vi "PRIME Detector Check Files and Add FITS data.vi"(5 "Observation":T2={"Priority"=0, "ID"="", "Observer"="", "Obj Name"="", "Obj Type"="", "RA and DEC String"={"RA"="HH:MM:SS.nnn", "DEC"="DEG:arcmin:arcsec.nn"}, "Filters"=[], "Integration Time"=0.0, "Observation Status"=enum."Error", "Offsets"={"RA"=0.0, "DEC"=0.0, "ROT"=0.0}, "Images"=0, "Dither Options"={"Dither"=enum."None", "Dither Radius"=0.0, "Dither Points"=0, "Dither Phase"=0.0, "B Offset"={"RA"=0.0, "DEC"=0.0}}, "Comment 1"="", "Comment 2"=""}, 7 "Detector Config":T8={"Detector"=0, "Offsets"=[[0, 0, 0, 0, 0, 0, 0, 0, 0, 0, 0, 0, 0, 0, 0, 0, 0, 0, 0, 0, 0, 0, 0, 0, 0, 0, 0, 0, 0, 0, 0, 0]], "Detector Computer"={"Machine"="192.168.121.11", "Password"="rSL!nux23456", "FITS File Path"="", "Port"=44444, "Header Path"="", "Name"=""}, "FITS hdr template0"=path "", "FITS hdr template1"=path "", "FITS Data File Path"=path "", "FITS Detector Settings"={"Exp Time Short"=0.0, "# of Frames"=0.0, "Exp Time Long"=0.0, "# of Groups"=0.0, "Object Name"="", "Object"="", "Obs Type"="", "Image Type"="", "Observer"="", "Observer Affiliation"=""}, "Sim Folder"=path "", "Integration Mode"=enum."Ramp", "Integration Time"=0.0, "Frame Int Time"=0.0} {"Offsets" format="%04x"; "Detector" items=["0", "1", "2"]}, 8 "error in (no error)":errorcluster, 9 "Image Type":string, 10 "Image Array":cluster{"CAMERA3":string[]}[](array[cluster]), 11 "Map in":map{string, T1}(c390)) -> (0 "error out":errorcluster, 3 "Map out":map{string, T1}(c390))   [LabVIEW 2024]
uses:
  RIMAS Detector Config.ctl
  RIMAS Detector Server Config.ctl
  RIMAS Observation Config.ctl
  Detector enum Detector Integration Mode.ctl
  typedefs/CC cluster Observation.ctl
  Observation Queue/CC enum Observation Status.ctl
  Telescope/CC cluster Telescope Offsets.ctl
  typedefs/CC cluster Observation Dither Options.ctl
  typedefs/CC enum Dither Selection.ctl
  typedefs/CC cluster RA and DEC.ctl
  Detector Image typedef cluster.ctl
  Detector Class.lvclass
panel:
  # "sec"
  # "sec"
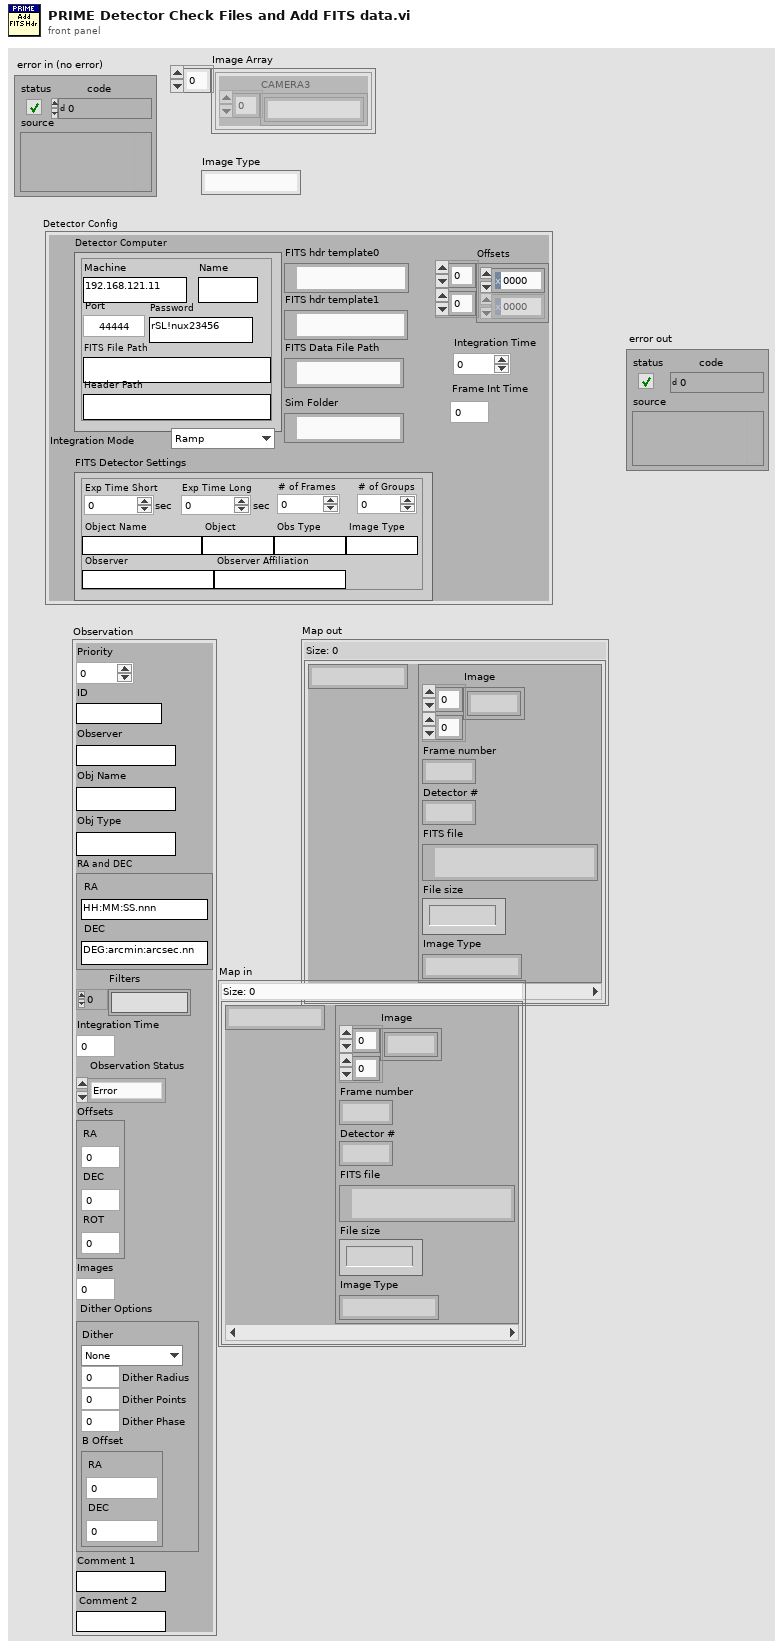
[diagram p1: front panel]
types:
  T1 = typedef "Detector Class.lvclass/Detector Image typedef cluster.ctl" = cluster{"Image":sgl[][], "Frame number":i32, "Detector #":u16, "FITS file":path, "File size":i64, "Image Type":string}
  T2 = typedef "CC cluster Observation.ctl" = cluster{"Priority":i32, "ID":string, "Observer":string, "Obj Name":string, "Obj Type":string, "RA and DEC String":cluster{"RA":string, "DEC":string}, "Filters":string[], "Integration Time":dbl, "Observation Status":T3, "Offsets":T4, "Images":i32, "Dither Options":T5, "Comment 1":string, "Comment 2":string}
  T3 = typedef "CC enum Observation Status.ctl" = enum16{"Ready", "Running", "Done", "Error"}
  T4 = typedef "CC cluster Telescope Offsets.ctl" = cluster{"RA":dbl, "DEC":dbl, "ROT":dbl}
  T5 = typedef "CC cluster Observation Dither Options.ctl" = cluster{"Dither":T6, "Dither Radius":dbl, "Dither Points":i32, "Dither Phase":dbl, "B Offset":T7}
  T6 = typedef "CC enum Dither Selection.ctl" = enum16{"None", "Circle", "Random", "ABBA"}
  T7 = typedef "CC cluster RA and DEC.ctl" = cluster{"RA":dbl, "DEC":dbl}
  T8 = typedef "RIMAS Detector Config.ctl" = cluster{"Detector":u16, "Offsets":u16[][], "Detector Computer":T9, "FITS hdr template0":path, "FITS hdr template1":path, "FITS Data File Path":path, "FITS Detector Settings":T10, "Sim Folder":path, "Integration Mode":T11, "Integration Time":dbl, "Frame Int Time":dbl}
  T9 = typedef "RIMAS Detector Server Config.ctl" = cluster{"Machine":string, "Password":string, "FITS File Path":string, "Port":u16, "Header Path":string, "Name":string}
  T10 = typedef "RIMAS Observation Config.ctl" = cluster{"Exp Time Short":dbl, "# of Frames":dbl, "Exp Time Long":dbl, "# of Groups":dbl, "Object Name":string, "Object":string, "Obs Type":string, "Image Type":string, "Observer":string, "Observer Affiliation":string}
  T11 = typedef "Detector enum Detector Integration Mode.ctl" = enum16{"Ramp", "CDS", "FOWLER2", "FOWLER4", "FOWLER8", "FOWLER16", "Raw"}
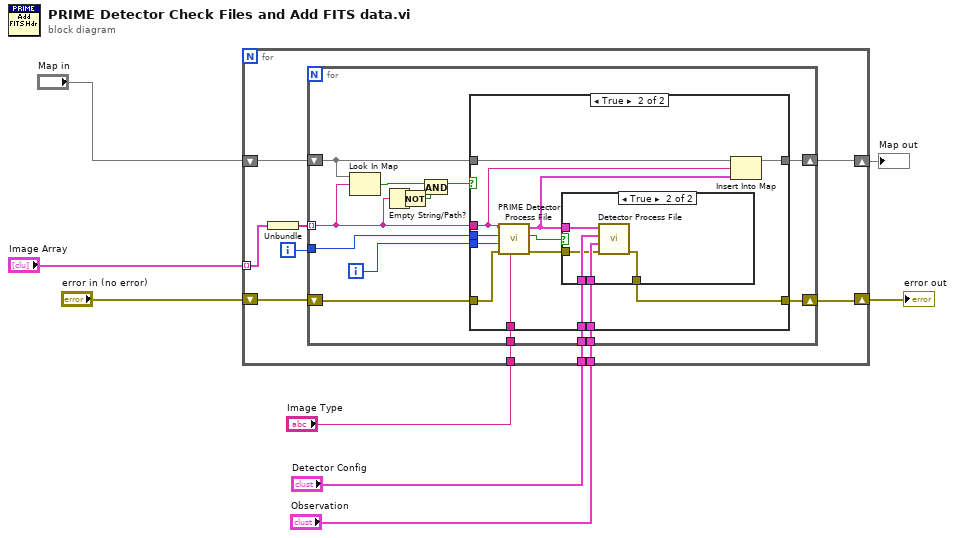
[diagram p0: block diagram]
diagram:
  n1 = for {
    shift-right: [w14] -> w4
    shift-left: "Map in" -> [w18]
    tunnel: "Image Array" -> [w17] mode=indexing
    tunnel: "Detector Config" -> [w13]
    tunnel: "Observation" -> [w12]
    shift-right: [w10] -> w2
    shift-left: "error in (no error)" -> [w11]
    tunnel: "Image Type" -> [w9]
    i -> [w15]
    n2 = Unbundle(w17) -> ("CAMERA3"=w16:string[])
    n3 = for {
      shift-right: [w28] -> w14
      shift-left: w18 -> [w29]
      tunnel: w16 -> [w23] mode=indexing
      tunnel: w15 -> [w31]
      tunnel: w13 -> [w27]
      tunnel: w12 -> [w26]
      shift-right: [w24] -> w10
      shift-left: w11 -> [w25]
      tunnel: w9 -> [w19]
      i -> [w30]
      n4 = Look In Map(map=w29, key=w23) -> (key not found?=w32:bool)  [unwired: 1 in, 1 out]
      n5 = Empty String/Path?(string/path=w23) -> (empty?=w21:bool)
      n6 = Not(x=w21) -> (.not. x?=w20:bool)
      n7 = And(x=w32, y=w20) -> (x .and. y?=w22:bool)
      n8 = case shown="True" w22 {
        tunnel: w23 -> [_ w44]
        tunnel: w31 -> [_ w47]
        tunnel: w30 -> [_ w46]
        tunnel: w29 -> [w34 w45]
        tunnel: [w34 w42] -> w28
        tunnel: w27 -> [_ w41]
        tunnel: w26 -> [_ w40]
        tunnel: w25 -> [w33 w39]
        tunnel: [w33 w37] -> w24
        tunnel: w19 -> [_ w35]
        frame False {
        }
        frame True {
          n9 = call "PRIME Detector Process File.vi"("Image Type"=w35, "error in (no error)"=w39, "Frame"=w46, "Camera"=w47, "Filename"=w44) -> ("error out"=w38:errorcluster, "Keep?"=w36:bool, "Image Data"=w43:T1)  [unwired: 4 in]
          n10 = case shown="True" w36 {
            tunnel: w43 -> [_ w53]
            tunnel: w41 -> [_ w52]
            tunnel: w40 -> [_ w51]
            tunnel: w38 -> [w48 w50]
            tunnel: [w48 w49] -> w37
            frame False {
            }
            frame True {
              n11 = call "Detector Process File.vi"("error in (no error)"=w50, "Observation"=w51, "Detector Config"=w52, "Image"=w53) -> ("error out"=w49:errorcluster)  [unwired: 6 in, 1 out]
            }
          }
          n12 = Insert Into Map(map in=w45, key=w44, value=w43) -> (map out=w42:map{string, T1})  [unwired: 2 out]
        }
      }
    }
  }
  "error out" <- w2
  "Map out" <- w4
